vi "Window Properties by Coef.vi"(11 "Window Coefficients":dbl[](array[numeric])) -> (0 "error":i32, 2 "coherent gain":dbl, 3 "eq noise BW":dbl)   [LabVIEW 2020, in "NI_AALPro.lvlib"]
doc: "Computes the coherent gain and equivalent noise bandwidth of a window. You must manually select the polymorphic instance you want to use."
uses:
  <vilib>/Analysis/NI_AALPro.lvlib
  <resource>/lvanlys.dll
panel:
  # "Window Properties"
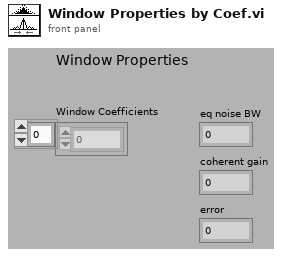
[diagram p1: front panel]
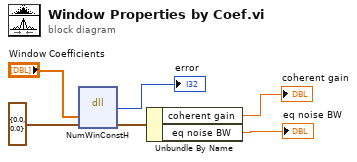
[diagram p0: block diagram]
diagram:
  n1 = dll-call lib="e:/builds/penguin/labview/branches/2020/dev/dist/resource/lvanlys.*" fn="NumWinConstH"("Window Coefficients"="Window Coefficients", "window constants"=cluster{"eq noise BW":dbl, "coherent gain":dbl} {"eq noise BW"=0.0, "coherent gain"=0.0}) -> (→"error":i32, "window constants"=w3:cluster{"eq noise BW":dbl, "coherent gain":dbl})  [unwired: 4 in, 2 out]
  n2 = Unbundle By Name(w3) -> ("coherent gain"=→"coherent gain":dbl, "eq noise BW"=→"eq noise BW":dbl)
